vi "replaceNodes.vi"(8 "error in (no error)":errorcluster, 9 "Replace Class":string, 10 "ToReplaceNode*":refnum<data-value>, 11 "RootNode* in":refnum<data-value>) -> (0 "error out":errorcluster, 2 "ReplaceNode*":refnum<data-value>, 3 "RootNode* out":refnum<data-value>)   [LabVIEW 2013, in "xceRootNode.lvclass"]
doc: "Replaces a node with another based of the class you wish to replace with. Used to swap out nodes"
uses:
  xceRootNode.lvclass
  xceDataNode/xceDataNode.lvclass
  xceRootNode.lvclass/xceRootNode.ctl
  xceNode/xceNode.lvclass
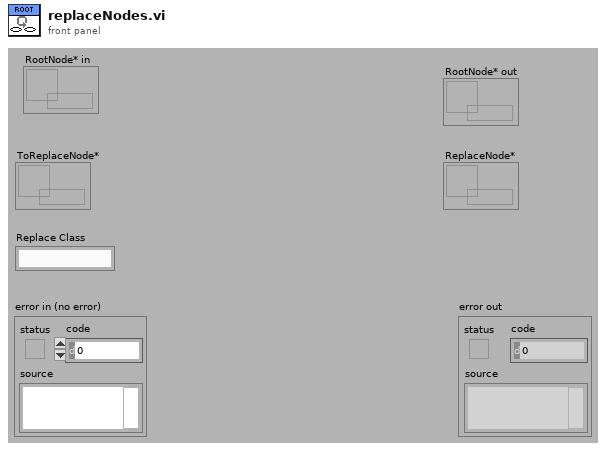
[diagram p1: front panel]
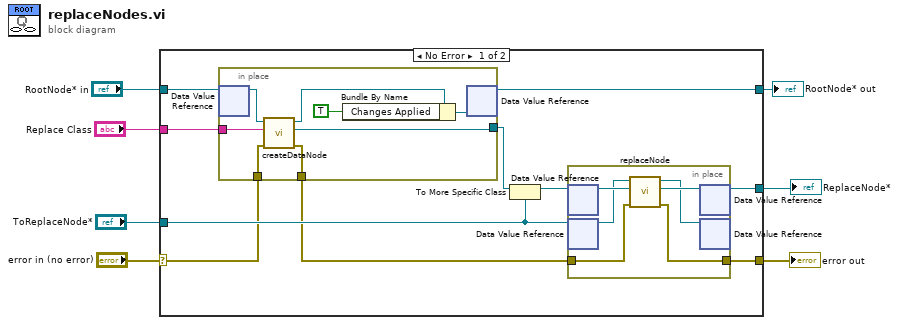
[diagram p0: block diagram]
diagram:
  n1 = case shown="No Error" "error in (no error)" {
    selector: "error in (no error)" -> [w12 w33]
    tunnel: [w9 w33] -> w6
    tunnel: "Replace Class" -> [w17 _]
    tunnel: "ToReplaceNode*" -> [w15 _]
    tunnel: "RootNode* in" -> [w16 w32]
    tunnel: [w10 w32] -> w1
    tunnel: [w8 _] -> w2
    frame No Error {
      n2 = in-place {
        in-place-border: w17 -> [w25]
        in-place-border: [w23] -> w14
        in-place-border: w12 -> [w22]
        in-place-border: [w21] -> w11
        n3 = in-place-dvr #1(w16) -> (w24:refnum<class "xceRootNode.lvclass">)  [unwired: 1 out]
        n4 = call "createDataNode.vi"("error in (no error)"=w22, "Data Class"=w25, "xceRootNode in"=w24) -> ("error out"=w21:errorcluster, "newNode*"=w23:refnum<data-value>, "xceRootNode out"=w20:refnum<class "xceRootNode.lvclass">)  [unwired: 6 in]
        n5 = Bundle By Name(cluster=w20, "Changes Applied"=TRUE) -> (w19:refnum<class "xceRootNode.lvclass">)
        n6 = in-place-dvr #1(w19) -> (w10:refnum<data-value>)  [unwired: 1 out]
      }
      n7 = To More Specific Class(target class=w15, reference=w14) -> (specific class reference=w13:refnum<data-value>)  [unwired: 1 in, 1 out]
      n8 = in-place {
        in-place-border: w11 -> [w27]
        in-place-border: [w26] -> w9
        n9 = in-place-dvr #2(w13) -> (w31:refnum<class "xceDataNode.lvclass">)  [unwired: 1 out]
        n10 = in-place-dvr #3(w15) -> (w29:refnum<class "xceDataNode.lvclass">)  [unwired: 1 out]
        n11 = call "replaceNode.vi"("error in (no error)"=w27, "ReplacerNode"=w31, "ReplaceNode"=w29) -> ("error out"=w26:errorcluster, "ReplacerNode out"=w30:refnum<class "xceDataNode.lvclass">, "ReplaceNode out"=w28:refnum<class "xceDataNode.lvclass">)  [unwired: 6 in]
        n12 = in-place-dvr #2(w30) -> (w8:refnum<data-value>)  [unwired: 1 out]
        n13 = in-place-dvr #3(w28) -> ()  [unwired: 2 out]
      }
    }
    frame Error {
    }
  }
  "error out" <- w6
  "ReplaceNode*" <- w2
  "RootNode* out" <- w1
